vi "sendToFPGA.vi"(8 "error in (no error)":errorcluster, 10 "Data":u16[](array[numeric]), 11 "Modbus in":refnum<class "Modbus.lvclass">) -> (0 "error out":errorcluster, 3 "Modbus out":refnum<class "Modbus.lvclass">)   [LabVIEW 2015, in "RTModbus.lvlib" / "Modbus.lvclass"]
uses:
  Modbus.lvclass
  Modbus.lvclass/Modbus.ctl
  Common_RT_FPGA/IWriteFIFO/IWriteFIFO.lvclass
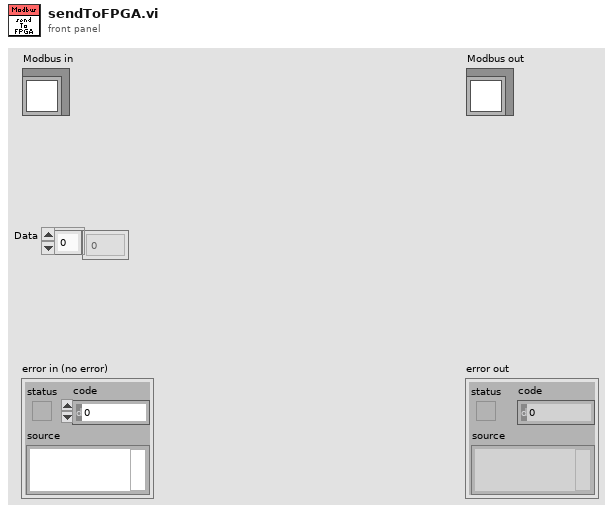
[diagram p1: front panel]
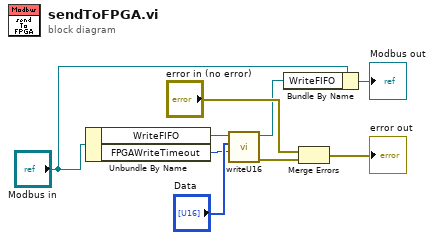
[diagram p0: block diagram]
diagram:
  n1 = Unbundle By Name("Modbus in") -> ("WriteFIFO"=w7:refnum<class "IWriteFIFO.lvclass">, "FPGAWriteTimeout"=w5:i32)
  n2 = call-dynamic "writeU16.vi"("Timeout"=w5, "Data"="Data", "IWriteFIFO in"=w7) -> ("error out"=w3:errorcluster, "IWriteFIFO out"=w1:refnum<class "IWriteFIFO.lvclass">)  [unwired: 6 in, 1 out]
  n3 = Bundle By Name(cluster="Modbus in", "WriteFIFO"=w1) -> (→"Modbus out":refnum<class "Modbus.lvclass">)
  n4 = Merge Errors("error in (no error)", w3) -> (→"error out":errorcluster)
